vi "getMagnetVector.vi"(8 "error in (no error)":errorcluster, 11 "Instrument.VRM in":refnum<class "Instrument.OxfordVRM.lvclass">) -> (0 "error out":errorcluster, 1 "status":string, 2 "Magnet Field (T)":dbl[](array[numeric]), 3 "Instrument.VRM out":refnum<class "Instrument.OxfordVRM.lvclass">, 4 "finished":bool)   [LabVIEW 2019, in "Instrument.OxfordVRM.lvclass"]
uses:
  Instrument.OxfordVRM.lvclass
  <userlib>/LevyLab/Instrument Framework/Instrument Types/Cryostat/Instrument.Cryostat.lvclass
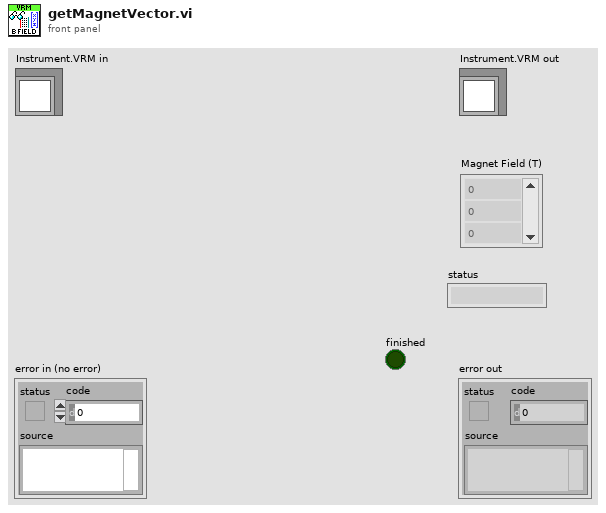
[diagram p1: front panel]
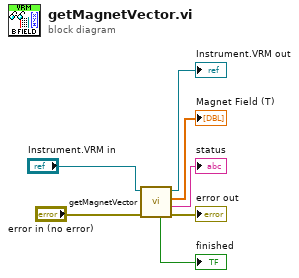
[diagram p0: block diagram]
diagram:
  n1 = call-parent "getMagnetVector.vi"("error in (no error)"="error in (no error)", "Instrument.Cryostat in"="Instrument.VRM in") -> ("error out"=→"error out":errorcluster, "Status"=→"status":string, "Field (T)"=→"Magnet Field (T)":dbl[], "Instrument.Cryostat out"=→"Instrument.VRM out":refnum<class "Instrument.OxfordVRM.lvclass">, "Finished?"=→"finished":bool)  [unwired: 5 in]
